vi "append_console_string.vi"(8 "error in (no error)":errorcluster, 9 "color":u32(colorbox), 10 "newline":string, 11 "console (in)":refnum<vi>) -> (0 "error out":errorcluster, 3 "reference out":refnum<vi>)   [LabVIEW 2021, in "console.provider.lvclass"]
uses:
  console.provider.lvclass
  console.provider.lvclass/console.provider.ctl
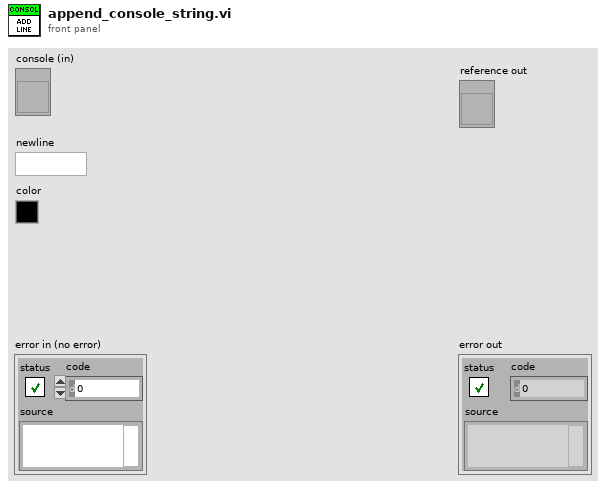
[diagram p1: front panel]
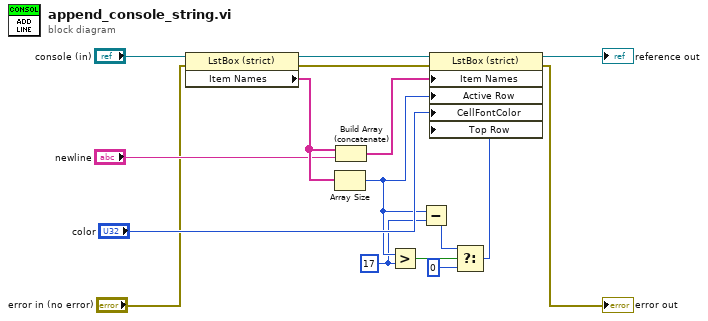
[diagram p0: block diagram]
diagram:
  w4 = 17 ("y")
  n1 = property class="LstBox (strict)"(reference="console (in)", error in="error in (no error)") -> (reference out=w13:refnum<vi>, error out=w8:errorcluster, "Item Names"=w15:string[])
  n2 = Array Size(array=w15) -> (size(s)=w5:i32)
  n3 = Build Array (concatenate)(w15, "newline") -> (w12:string[])
  n4 = Greater?(x=w5, y=w4) -> (0:w6:bool)
  n5 = Subtract(x=w5, y=w4) -> (x-y=w3:i32)
  n6 = Select(t=w3, s=w6, f=0) -> (s? t:f=w1:i32)
  n7 = property class="LstBox (strict)"(reference=w13, error in=w8, "Item Names"=w12, "Active Row"=w5, "CellFontColor"="color", "Top Row"=w1) -> (reference out=→"reference out":refnum<vi>, error out=→"error out":errorcluster)
